vi "STAGE+mono+counter_edit13.vi"() -> ()   [LabVIEW 2017]
panel:
  out "XY Graph 2":cluster{"X":dbl, "Y":dbl}[](graph)
  out "Numeric 2":i32
  out "Numeric":i32
  out "?":cluster{dbl[], dbl[]}(graph)
  out "XY Graph":cluster{dbl[], dbl[]}(graph)
  out "Slide":u8(slide) max=10 step=10 scale=0.0..10.0
  in  "?":enum32{"DELAY", "COUNTER", "MONO", "PLOT"}(tab)
  out "Final time [ps]":dbl
  out "Current time [ps]":dbl
  out "Initial time [ps]":dbl
  in  "Set this as t0":bool
  in  "Axis":i32=1
  in  "Motor ON":bool
  in  "Motor OFF":bool
  out "Current Position [mm]":dbl
  out "Final Position [mm]":dbl
  in  "Data Points":i32=100
  out "Current Point":i32
  in  "Step Size [um]":i32=10
  in  "Target [mm]":dbl format="%.3f"
  in  "Move":bool
  out "Initial position [mm]":dbl
  in  "GPIB address":string="23"
  in  "Count Mode":u16(ring) items=["A,B for Preset T", "A-B for Preset T", "A+B for Preset T", "A for Preset B"]
  in  "Trigger mode":u16(ring) items=["10 MHz"=0, "Input 2"=2, "Input T"=3]
  in  "Channel A Input":u16(ring)=1 items=["10 MHz", "Input 1"]
  in  "Channel B Input":u16(ring)=2 items=["Input 1"=1, "Input 2"=2]
  in  "Number of Measurements\n to take at one point/ Number of Periods":u16=1 min=1 max=2000 step=1
  in  "Time between measurements\n at one point (s)/Dwell Time":dbl=0.002 min=0.002 max=60.0 step=0.001
  in  "gate A mode (CW:0)":i16(slide) scale=0.0..2.0 scale format="%.2f"
  out "Counts":i32
  in  "Integrating time, 10^-7 sec":dbl=10000000.0
  out "Mono port":T1(ring)
  out "Time delay":u32=450000 min=1
  out "Serial":u32=12345
  in  "Step size":dbl=10.0 min=0.0
  in  "Scan to":i32=4000
  in  "Scan from":i32=2600
  out "Current wavelength":dbl
  out "Grt#":u8=1 min=1 max=3 step=1
  in  "?":bool
  out "Groove/mm":u32=1200
  out "Blaze (nm)":u32=300
  in  "Array":dbl[](array[numeric])
  out "Timeout 2":bool
  in  "?":bool
  out "Timeout":bool
  in  "Collect Data!":bool
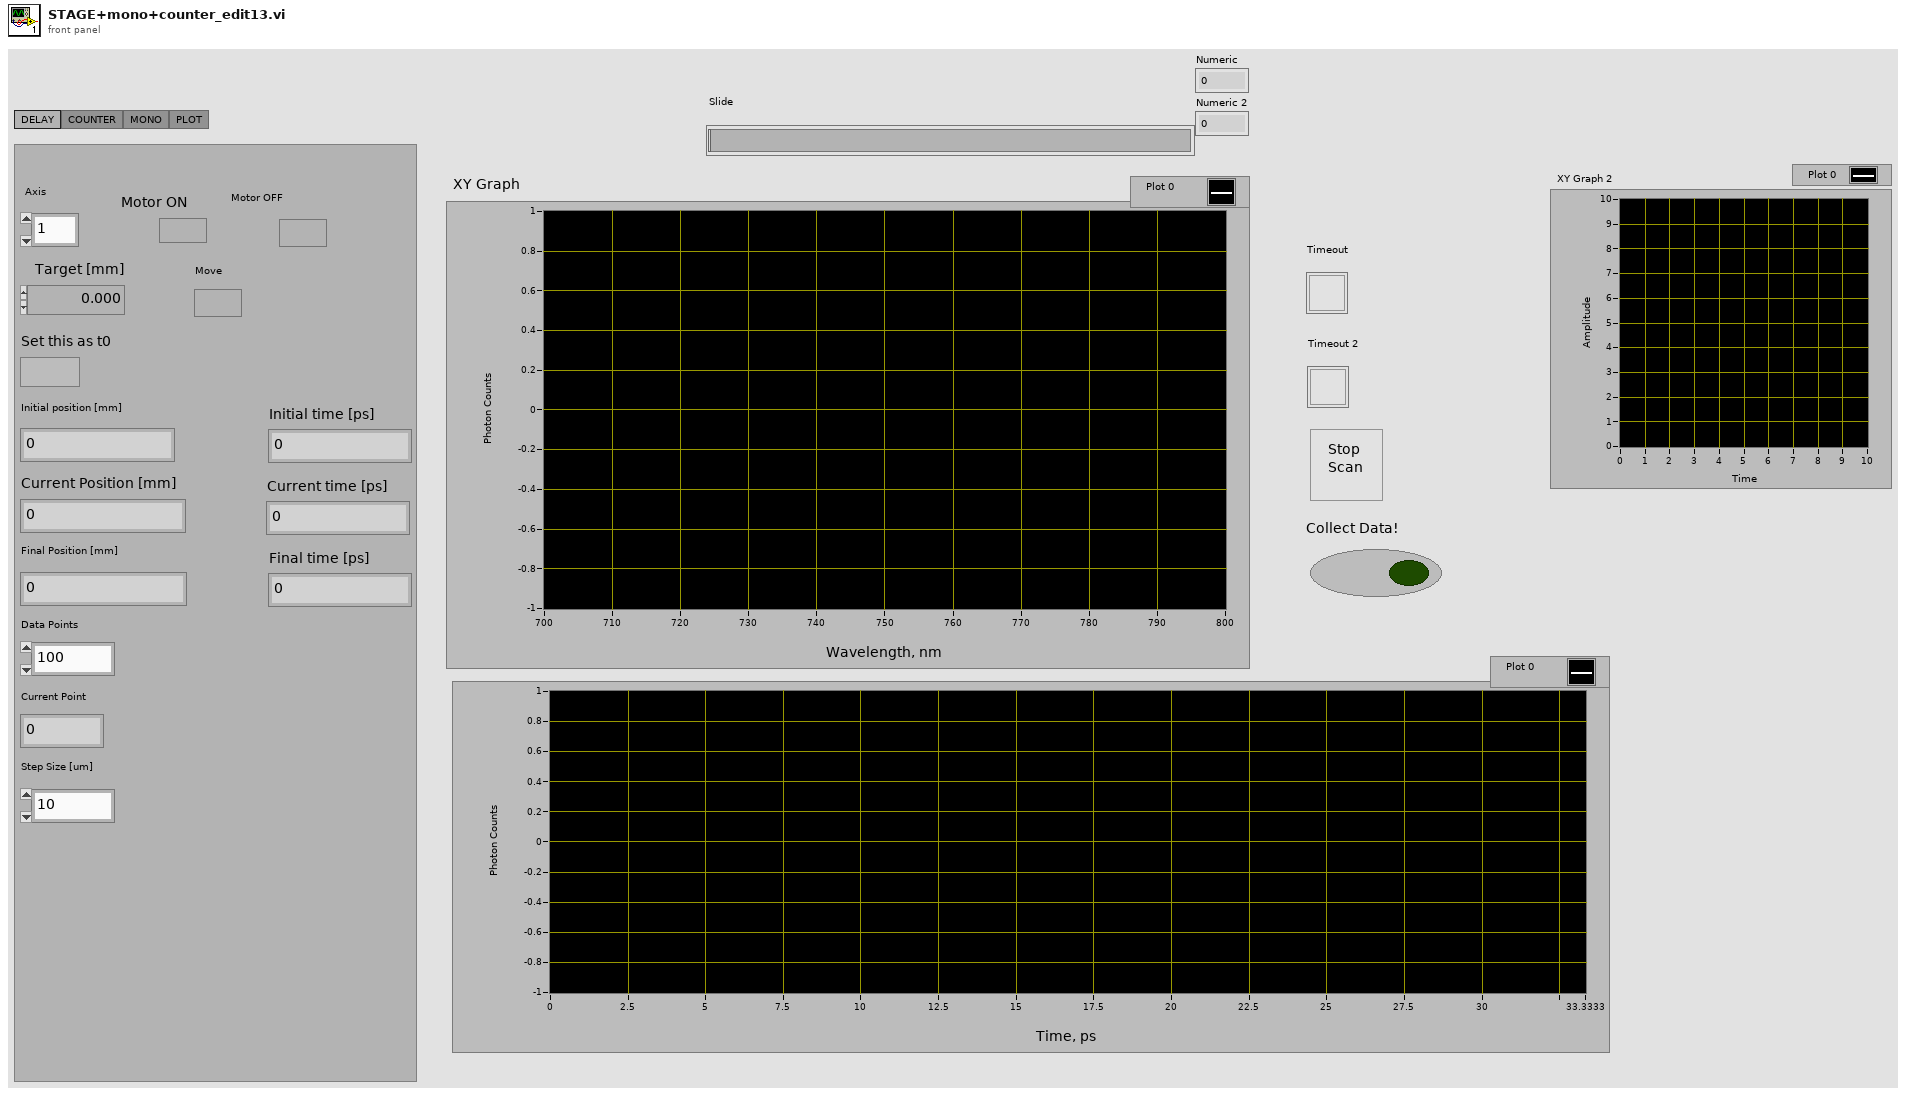
[diagram p1: front panel]
types:
  T1 = enum8{"COM 1", "COM 2", "COM 3", "COM 4", "COM 5", "COM 6", "COM 7", "COM 8", "COM 9"}
  T2 = cluster{"input XON/XOFF":bool, "input HW Handshake":bool, "input alt HW HShk":bool, "output XON/XOFF":bool, "output HW Handshake":bool, "output alt HW HShk":bool, "XOFF byte":u8, "XON byte":u8, "parity error byte":u16}
  T3 = enum16{"no parity", "odd parity", "even parity", "mark parity", "space parity"}
  T4 = cluster{"Y[0]":dbl, "Y[1]":dbl, "Y[2]":dbl, "Y[3]":dbl, "Y[4]":dbl, "Y[5]":dbl, "Y[6]":dbl, "Y[7]":dbl, "Y[8]":dbl}
  T5 = typedef "NI_Matrix.lvlib/RealMatrix.ctl" = dbl[][]
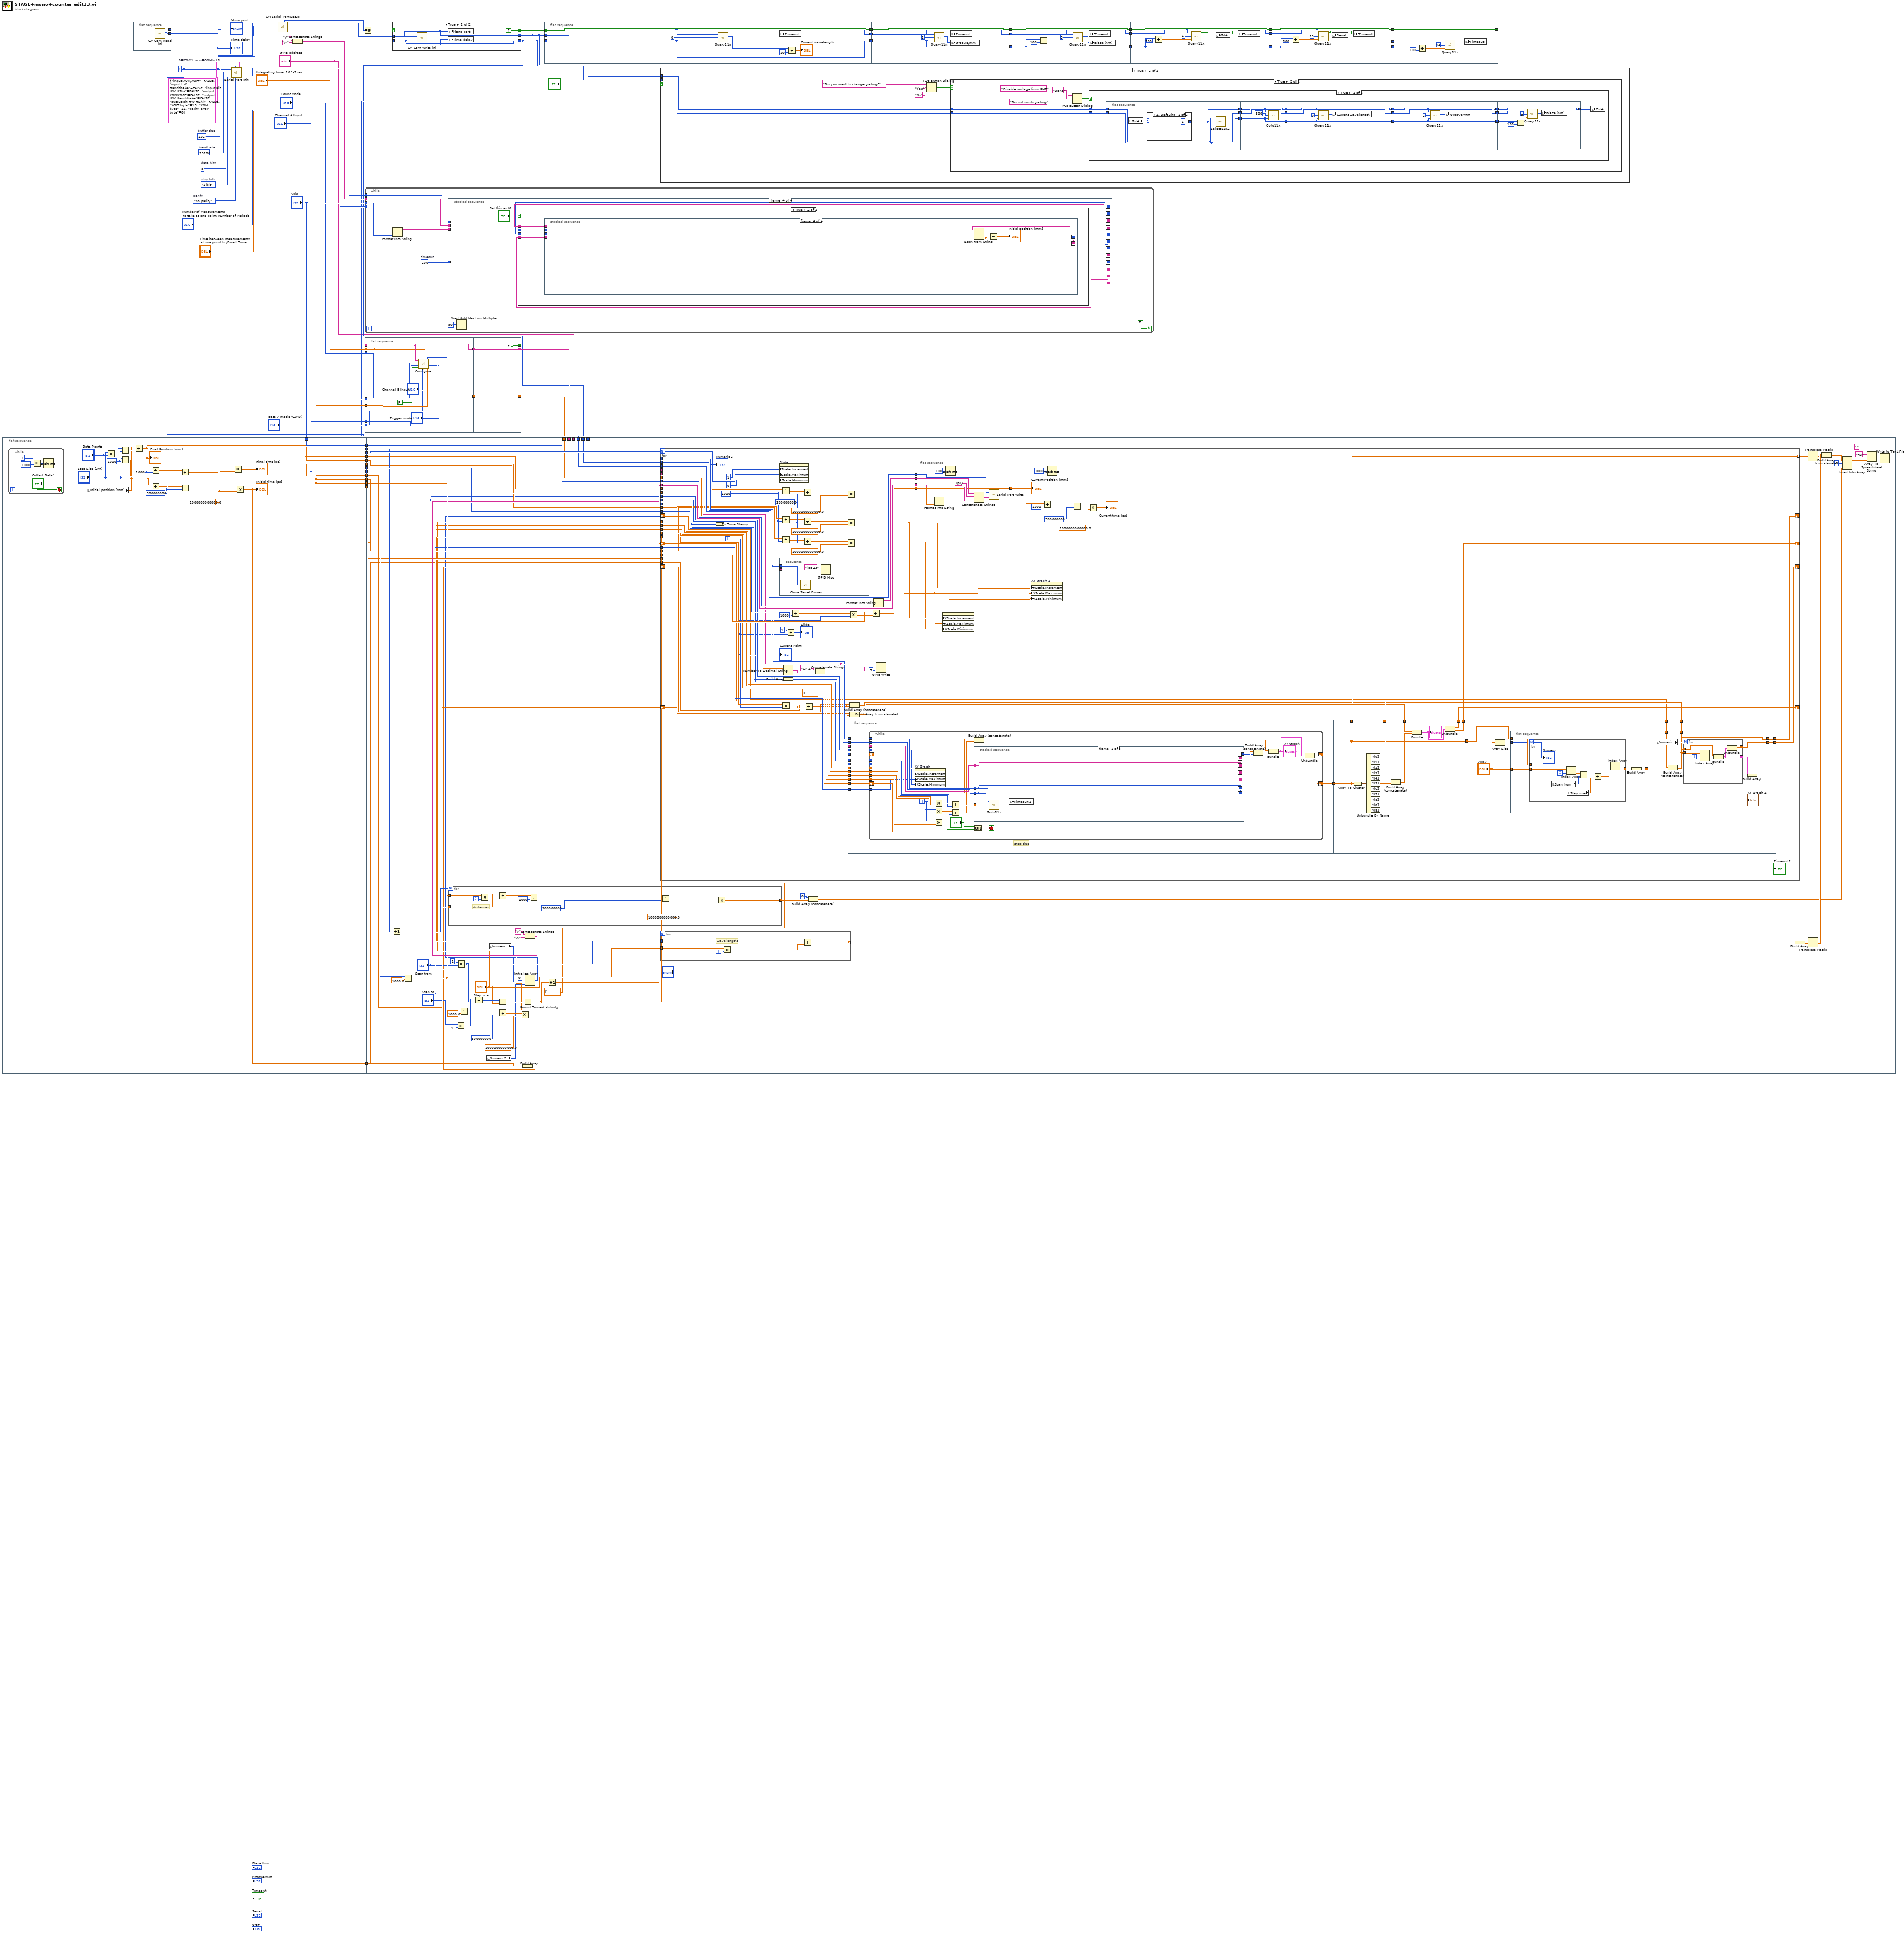
[diagram p0: block diagram]
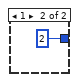
[diagram p5: hidden frame]
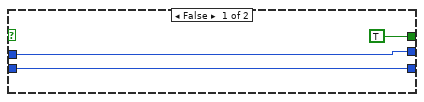
[diagram p6: hidden frame]
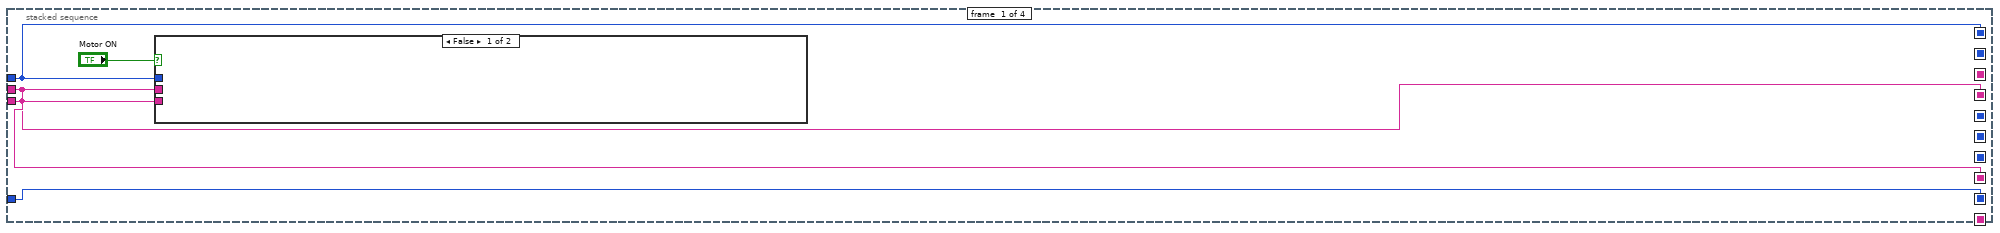
[diagram p7: hidden frame]
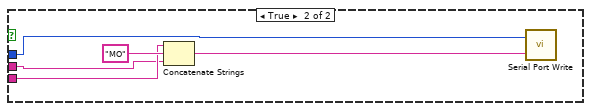
[diagram p8: hidden frame]
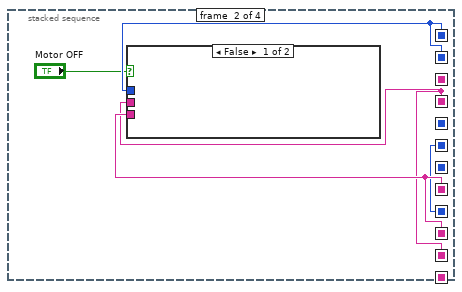
[diagram p9: hidden frame]
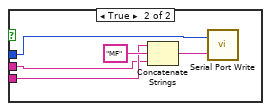
[diagram p10: hidden frame]
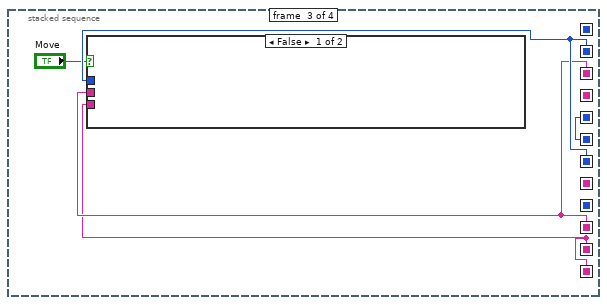
[diagram p11: hidden frame]
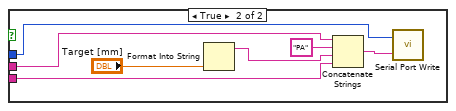
[diagram p12: hidden frame]
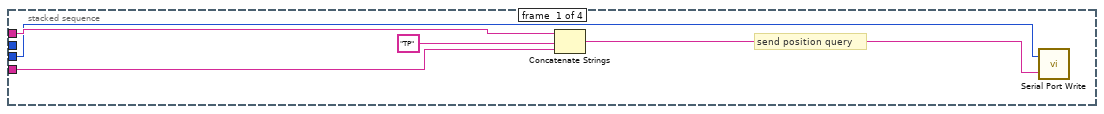
[diagram p14: hidden frame]
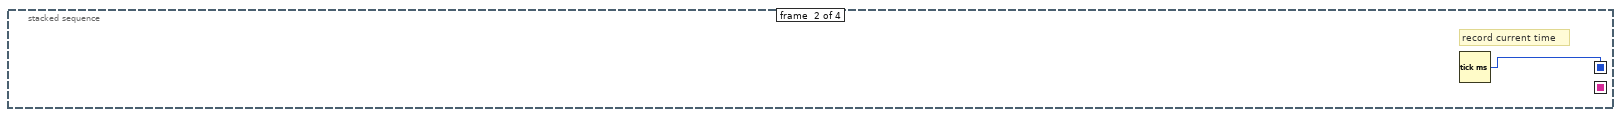
[diagram p15: hidden frame]
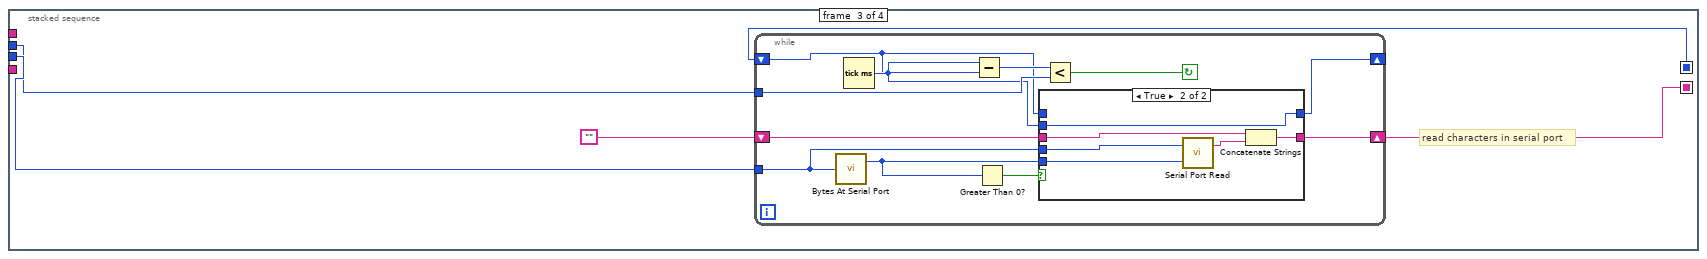
[diagram p16: hidden frame]
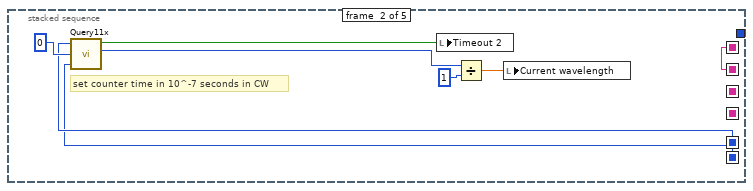
[diagram p18: hidden frame]
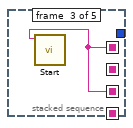
[diagram p19: hidden frame]
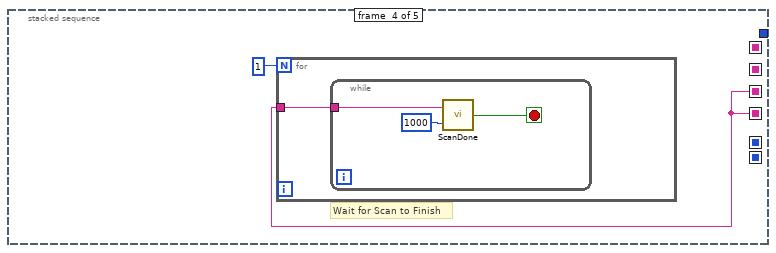
[diagram p20: hidden frame]
diagram:
  w55 = u32 19200  # baud rate
  w54 = u16 8  # data bits
  w53 = enum16{"1 bit", "1.5 bits", "2 bits"}."1 bit"  # stop bits
  w57 = T3."no parity"  # parity
  w52 = 4  # 0=COM1 so n=COM(n+1)
  w56 = u16 1024  # buffer size
  n1 = flat-sequence {
    tunnel: ["Data Points"] -> w61
    tunnel: "Axis" -> [w83]
    tunnel: [w75] -> w60
    tunnel: [w83] -> w59
    tunnel: ["Step Size [um]"] -> w12
    tunnel: [w75] -> w11
    tunnel: ["Step Size [um]"] -> w10
    tunnel: ["Data Points"] -> w9
    tunnel: [w75] -> w8
    tunnel: [w74] -> w7
    tunnel: [w75] -> w4
    tunnel: [w74] -> w3
    tunnel: [w77] -> w2
    tunnel: [w67] -> w1
    tunnel: w61 -> [w145]
    tunnel: w60 -> [w144]
    tunnel: w59 -> [w143]
    tunnel: w52 -> [w139]
    tunnel: w16 -> [w138]
    tunnel: w15 -> [w137]
    tunnel: w14 -> [w136]
    tunnel: "GPIB address" -> [w135]
    tunnel: w12 -> [w122]
    tunnel: w11 -> [w120]
    tunnel: w10 -> [w119]
    tunnel: w9 -> [w117]
    tunnel: w8 -> [w110]
    tunnel: w7 -> [w109]
    tunnel: w6 -> [w108]
    tunnel: w4 -> [w106]
    tunnel: w3 -> [w105]
    tunnel: w2 -> [w104]
    tunnel: w1 -> [w102]
    frame #0 {
      n2 = while {
        stop <- "Collect Data!" stop-if-true
        n3 = Multiply(x=1, y=1000) -> (x*y=w65:i32)
        n4 = Wait (ms)(milliseconds to wait=w65) -> ()  [unwired: 1 out]
      }
    }
    frame #1 {
      w68 = 1000000000000.0
      w73 = 1000
      w76 = 300000000
      w78 = 1000
      n5 = local read "Initial position [mm]"() -> (w75:dbl)
      n6 = Multiply(x="Step Size [um]", y="Data Points") -> (x*y=w82:i32)
      n7 = Divide(x=w82, y=w78) -> (x/y=w81:dbl)
      n8 = Divide(x="Step Size [um]", y=w78) -> (x/y=w77:dbl)
      n9 = Add(x=w75, y=w81) -> (x+y=w74:dbl)
      "Final Position [mm]" <- w74
      n10 = Divide(x=w74, y=w73) -> (x/y=w72:dbl)
      n11 = Divide(x=w75, y=w73) -> (x/y=w71:dbl)
      n12 = Divide(x=w72, y=w76) -> (x/y=w69:dbl)
      n13 = Divide(x=w71, y=w76) -> (x/y=w70:dbl)
      n14 = Multiply(x=w69, y=w68) -> (x*y=→"Final time [ps]":dbl)
      n15 = Multiply(x=w70, y=w68) -> (x*y=w67:dbl)
      "Initial time [ps]" <- w67
    }
    frame #2 {
      n16 = Increment(x=w117) -> (x+1=w118:i32)
      n17 = Divide(x=w122, y=1000.0) -> (x/y=w96:dbl)
      n18 = for {
        N: w118 -> [_]
        tunnel: w96 -> [w156]
        tunnel: w120 -> [w154]
        tunnel: [w147] -> w116 mode=indexing
        i -> [w155]
        # "distances"
        n19 = Multiply(x=w156, y=w155) -> (x*y=w153:dbl)
        n20 = Add(x=w154, y=w153) -> (x+y=w152:dbl)
        n21 = Divide(x=w152, y=1000) -> (x/y=w146:dbl)
        n22 = Divide(x=w146, y=300000000) -> (x/y=w149:dbl)
        n23 = Multiply(x=w149, y=1000000000000.0) -> (x*y=w147:dbl)
      }
      n24 = Multiply(x="Scan to", y=1) -> (x*y=w103:i32)
      n25 = Multiply(x=1, y="Scan from") -> (x*y=w92:i32)
      n26 = Divide(x=w96, y=1000.0) -> (x/y=w97:dbl)
      n27 = Subtract(x=w103, y=w92) -> (x-y=w130:i32)
      n28 = local read "Numeric 2"() -> (w85:i32)
      n29 = local read "Numeric"() -> (w84:i32)
      n30 = Divide(x=w130, y="Step size") -> (x/y=w129:dbl)
      n31 = Divide(x=w97, y=300000000) -> (x/y=w99:dbl)
      n32 = Multiply(x=w99, y=1000000000000.0) -> (x*y=w95:dbl)
      n33 = Build Array(w102) -> (w89:dbl[])
      n34 = Round Toward -Infinity(1:w129) -> (0:w128:dbl)
      n35 = Concatenate Strings("\r", "\n") -> (w140:string)
      n36 = Initialize Array(0, w84, w85) -> (w87:i32[][])
      n37 = Increment(x=w128) -> (x+1=w91:dbl)
      n38 = for {
        N: w145 -> [w204]
        tunnel: w144 -> [w231]
        tunnel: w119 -> [w227]
        tunnel: w143 -> [w224]
        tunnel: w140 -> [w221]
        tunnel: w139 -> [w222]
        tunnel: w138 -> [w220]
        tunnel: w137 -> [w217]
        tunnel: w136 -> [w219]
        tunnel: w135 -> [w218]
        tunnel: [w169] -> w125 mode=indexing
        tunnel: w92 -> [w212]
        tunnel: "Step size" -> [w211]
        tunnel: w128 -> [w210]
        tunnel: w110 -> [_]
        tunnel: w109 -> [_]
        tunnel: w108 -> [w209]
        tunnel: "Scan to" -> [w208]
        tunnel: "Scan from" -> [w207]
        tunnel: "Step size" -> [w178]
        tunnel: w106 -> [w199]
        tunnel: w105 -> [w197]
        tunnel: w104 -> [w200]
        tunnel: w95 -> [w187]
        shift-right: [w171] -> _
        shift-left: w89 -> [w181]
        shift-right: [w170] -> _
        shift-left: dbl[] [] ("Y") -> [w176]
        tunnel: w102 -> [w205]
        tunnel: "Scan from" -> [w179]
        tunnel: "Step size" -> [w180]
        shift-right: [w168] -> _
        shift-left: w89 -> [w174]
        shift-right: [w166] -> _
        shift-left: w87 -> [w165]
        i -> [w186]
        w198 = 1000
        w201 = 300000000
        n39 = To Time Stamp(1:w212) -> ()  [unwired: 1 out]
        n40 = property on="Slide" class="Slide (strict)"("Scale.Increment"=1, "Scale.Maximum"=w204, "Scale.Minimum"=0) -> ()  [unwired: 2 in, 2 out]
        n41 = stacked-sequence {
          tunnel: w217 -> [w345]
          tunnel: w218 -> [_]
          frame #0 {
            n42 = call <vilib>:"Close Serial Driver.vi"("port number"=w345) -> ()  [unwired: 1 out]
            n43 = GPIB Misc(0:"loc 23" ("command string")) -> ()  [unwired: 1 in, 3 out]
          }
        }
        n44 = Divide(x=w197, y=w198) -> (x/y=w194:dbl)
        n45 = Divide(x=w200, y=w198) -> (x/y=w196:dbl)
        n46 = Divide(x=w199, y=w198) -> (x/y=w195:dbl)
        n47 = Multiply(x=w187, y=w186) -> (x*y=w206:dbl)
        n48 = Number To Decimal String(number=w209) -> (decimal integer string=w215:string)  [unwired: 1 in]
        n49 = Build Array(w179) -> (w183:i32[])
        n50 = Add(x=1, y=w186) -> (x+y=→"Slide":i32)
        n51 = Divide(x=w227, y=1000) -> (x/y=w226:dbl)
        n52 = Divide(x=w194, y=w201) -> (x/y=w188:dbl)
        n53 = Divide(x=w196, y=w201) -> (x/y=w190:dbl)
        n54 = Divide(x=w195, y=w201) -> (x/y=w189:dbl)
        n55 = Add(x=w205, y=w206) -> (x+y=w175:dbl)
        n56 = Concatenate Strings("CP 2,", w215) -> (w213:string)
        n57 = Multiply(x=w188, y=1000000000000.0) -> (x*y=w163:dbl)
        n58 = Multiply(x=w190, y=1000000000000.0) -> (x*y=w164:dbl)
        n59 = Multiply(x=w189, y=1000000000000.0) -> (x*y=w162:dbl)
        n60 = flat-sequence {
          tunnel: w220 -> [w245]
          tunnel: w219 -> [w244]
          tunnel: w217 -> [w243]
          tunnel: w212 -> [w242]
          tunnel: w211 -> [w241]
          tunnel: w210 -> [w240]
          tunnel: w208 -> [w239]
          tunnel: w207 -> [w238]
          tunnel: w183 -> [w237]
          tunnel: dbl[] [] ("Y") -> [w236]
          tunnel: w180 -> [w235]
          tunnel: w179 -> [w234]
          tunnel: w178 -> [w233]
          tunnel: [w232] -> w177
          tunnel: w177 -> [w299]
          tunnel: w176 -> [w306]
          tunnel: [w299] -> w173
          tunnel: w172 -> [w303]
          tunnel: [w301] -> w171
          tunnel: [w300] -> w170
          tunnel: [w299] -> w169
          tunnel: w173 -> [w315]
          tunnel: [w308] -> w168
          tunnel: w167 -> [w309]
          tunnel: w165 -> [w312]
          tunnel: [w310] -> w166
          frame #0 {
            # "step size"
            n61 = while {
              tunnel: w243 -> [w271]
              tunnel: w244 -> [w270]
              tunnel: w245 -> [w266]
              tunnel: w242 -> [w264]
              tunnel: w241 -> [w263]
              tunnel: w240 -> [w262]
              tunnel: w239 -> [w246]
              tunnel: w238 -> [w247]
              tunnel: w233 -> [w248]
              tunnel: w235 -> [w260]
              shift-right: [w255] -> w232
              shift-left: w236 -> [w254]
              shift-right: [w249] -> _
              shift-left: w237 -> [w258]
              tunnel: w234 -> [w252]
              i -> [w261]
              stop <- w269 stop-if-true
              n62 = property on="XY Graph" class="XYGraph (strict)"("XScale.Increment"=w248, "XScale.Maximum"=w246, "XScale.Minimum"=w247) -> ()  [unwired: 2 in, 2 out]
              n63 = Multiply(x=w261, y=w263) -> (x*y=w272:dbl)
              n64 = Multiply(x=w261, y=w260) -> (x*y=w259:dbl)
              n65 = Greater Or Equal?(x=w261, y=w262) -> (x >= y?=w267:bool)
              n66 = Add(x=w272, y=w264) -> (x+y=w265:dbl)
              n67 = Add(x=w259, y=w252) -> (x+y=w257:dbl)
              n68 = Or(x="?", y=w267) -> (x .or. y?=w269:bool)
              n69 = Build Array (concatenate)(w258, w257) -> (w256:dbl[])
              n70 = stacked-sequence {
                seq-local: [w276 _ _ _ _] -> [_ w284 _ _ _]
                seq-local: [w275 _ _ _ _] -> [_ w283 _ _ _]
                seq-local: [w273 _ _ _ _] -> [_ w281 _ _ _]
                seq-local: [_ w281 _ _ _] -> [_ _ w286 _ _]
                seq-local: [_ _ w286 _ _] -> [_ _ _ w287 _]
                seq-local: [_ _ _ w287 _] -> [_ _ _ _ w294]
                tunnel: w265 -> [w277 _ _ _ _]
                tunnel: w271 -> [w276 _ _ _ _]
                tunnel: w270 -> [w275 _ _ _ _]
                tunnel: w266 -> [w273 _ _ _ _]
                tunnel: [_ _ _ _ w293] -> w251
                frame #0 {
                  n71 = call "Goto11x.vi"("time delay"=w275, "WAVELENGTH"=w277, "port number"=w276) -> ("timeout"=w274:bool)  [unwired: 2 out]
                  n72 = local write "Timeout 2"(w274) -> ()
                }
                frame #1 {
                  # "set counter time in 10^-7 seconds in CW"
                  n73 = call "Query11x.vi"("port number"=w284, "QUERY"=0, "time delay"=w283) -> ("timeout"=w282:bool, "STATUS MESSAGE"=w280:u16)  [unwired: 2 out]
                  n74 = local write "Timeout 2"(w282) -> ()
                  n75 = Divide(x=w280, y=1) -> (x/y=w279:dbl)
                  n76 = local write "Current wavelength"(w279) -> ()
                }
                frame #2 {
                  n77 = call "Start.vi"("GPIB Address"=w286) -> ()  [unwired: 9 in]
                }
                frame #3 {
                  # "Wait for Scan to Finish"
                  n78 = for {
                    N: 1 -> [_]
                    tunnel: w287 -> [w289]
                    n79 = while {
                      tunnel: w289 -> [w290]
                      stop <- w292 stop-if-true
                      n80 = call "ScanDone.vi"("Wait (ms)"=1000, "GPIB Address"=w290) -> ("Scan Finished?"=w292:bool)
                    }
                  }
                }
                frame #4 {
                  n81 = call "Read Data.vi"("Channel Number"=0, "GPIB Address"=w294, "Number of Datapoints"=1) -> ("Data"=w295:i32[])
                  n82 = Index Array(array=w295, index=0) -> (element=w293:i32)
                  "Counts" <- w293
                }
              }
              n83 = Build Array (concatenate)(w254, w251) -> (w253:dbl[])
              n84 = Bundle(w256, w253) -> (w250:cluster{dbl[], dbl[]})  [unwired: 1 in]
              "XY Graph" <- w250
              n85 = Unbundle(w250) -> (w249:dbl[], w255:dbl[])
            }
          }
          frame #1 {
            n86 = Array To Cluster(array=w299) -> (cluster=w307:T4)
            n87 = Unbundle By Name(w307) -> ("Y[5]"=w305:dbl)  [unwired: 10 out]
            n88 = Build Array (concatenate)(w306, w305) -> (w304:dbl[])
            n89 = Bundle(w303, w304) -> (w302:cluster{dbl[], dbl[]})  [unwired: 1 in]
            "?" <- w302
            n90 = Unbundle(w302) -> (w301:dbl[], w300:dbl[])
          }
          frame #2 {
            n91 = Array Size(array="Array") -> (size(s)=w313:i32)
            n92 = flat-sequence {
              tunnel: w315 -> [w320]
              tunnel: "Array" -> [w319]
              tunnel: w313 -> [w318]
              tunnel: [w316] -> w311
              tunnel: w312 -> [w337]
              tunnel: w311 -> [w336]
              tunnel: [w334] -> w310
              tunnel: w309 -> [w333]
              tunnel: [w332] -> w308
              frame #0 {
                n93 = for {
                  N: w318 -> [w322]
                  tunnel: w319 -> [w330]
                  tunnel: w320 -> [w324]
                  tunnel: [w321] -> w317
                  i -> [w329]
                  n94 = local read "Scan from"() -> (w327:i32)
                  n95 = Index Array(array=w330, index=w329) -> (element=w328:dbl)
                  n96 = local read "Step size"() -> (w325:dbl)
                  n97 = Subtract(x=w328, y=w327) -> (x-y=w326:dbl)
                  n98 = Divide(x=w326, y=w325) -> (x/y=w323:dbl)
                  n99 = Index Array(array=w324, index=w323) -> (element=w321:dbl)
                  "Numeric" <- w322
                }
                n100 = Build Array(w317) -> (w316:dbl[])
              }
              frame #1 {
                n101 = local read "Numeric"() -> (w335:i32)
                n102 = Build Array (concatenate)(w337, w336) -> (w334:dbl[][])
                n103 = for {
                  N: w335 -> [_]
                  tunnel: w334 -> [w343]
                  tunnel: w333 -> [w341]
                  tunnel: [w340] -> w332
                  tunnel: [w338] -> w331 mode=indexing
                  i -> [w342]
                  n104 = Index Array(array=w343, index (row)=w342) -> (element=w339:dbl[])  [unwired: 1 in]
                  n105 = Bundle(w341, w339) -> (w338:cluster{dbl[], dbl[]})  [unwired: 1 in]
                  n106 = Unbundle(w338) -> (w340:dbl[])  [unwired: 1 out]
                }
                n107 = Build Array(w331) -> ()  [unwired: 1 out]
              }
            }
          }
        }
        n108 = Multiply(x=w226, y=w186) -> (x*y=w230:dbl)
        n109 = Build Array (concatenate)(w174, w175) -> (w167:dbl[])
        n110 = Build Array (concatenate)(w181, w175) -> (w172:dbl[])
        n111 = Add(x=w231, y=w230) -> (x+y=w229:dbl)
        n112 = Format Into String(w224) -> (resulting string=w223:string)  [unwired: 3 in, 1 out]
        n113 = GPIB Write(0:w220, 1:w213, 2:i16 5 ("mode (0)")) -> ()  [unwired: 2 in, 2 out]
        n114 = flat-sequence {
          tunnel: w229 -> [w348]
          tunnel: [w348] -> w225
          tunnel: w221 -> [w350]
          tunnel: w223 -> [w349]
          tunnel: w222 -> [w346]
          tunnel: w225 -> [w359]
          frame #0 {
            n115 = Format Into String(w348) -> (resulting string=w347:string)  [unwired: 3 in, 1 out]
            n116 = Wait (ms)(milliseconds to wait=u32 100) -> ()  [unwired: 1 out]
            n117 = Concatenate Strings(w349, "PA" ("Substring"), w347, w350) -> (w352:string)
            n118 = call <vilib>:"Serial Port Write.vi"("string to write"=w352, "port number"=w346) -> ()  [unwired: 1 out]
          }
          frame #1 {
            n119 = Divide(x=w359, y=1000) -> (x/y=w357:dbl)
            n120 = Wait (ms)(milliseconds to wait=u32 1000) -> ()  [unwired: 1 out]
            n121 = Divide(x=w357, y=300000000) -> (x/y=w356:dbl)
            n122 = Multiply(x=w356, y=1000000000000.0) -> (x*y=→"Current time [ps]":dbl)
            "Current Position [mm]" <- w359
          }
        }
        n123 = property class="XYGraph (strict)"("XScale.Increment"=w164, "XScale.Maximum"=w163, "XScale.Minimum"=w162) -> ()  [unwired: 2 in, 2 out]
        n124 = property on="XY Graph 2" class="XYGraph (strict)"("XScale.Increment"=w164, "XScale.Maximum"=w163, "XScale.Minimum"=w162) -> ()  [unwired: 2 in, 2 out]
        "Current Point" <- w186
        "Numeric 2" <- w204
      }
      n125 = for {
        N: w91 -> [_]
        tunnel: "Step size" -> [w161]
        tunnel: w92 -> [w159]
        tunnel: [w157] -> w90 mode=indexing
        i -> [w160]
        # "wavelengths"
        n126 = Multiply(x=w161, y=w160) -> (x*y=w158:dbl)
        n127 = Add(x=w159, y=w158) -> (x+y=w157:dbl)
      }
      n128 = Build Array (concatenate)(0, w116) -> (w113:dbl[])
      n129 = Build Array(w90) -> (w126:dbl[][])
      n130 = Transpose Matrix(1:w125) -> (0:w123:dbl[][])
      n131 = Transpose Matrix(1:w126) -> (0:w124:dbl[][])
      n132 = Build Array (concatenate)(w124, w123) -> (w112:T5)
      n133 = Insert Into Array(array=w112, index (row)=0, new element=w113) -> (w111:T5)  [unwired: 1 in]
      n134 = Array To Spreadsheet String(delimiter (Tab)=",", array=w111, 3:"%f" ("format string")) -> (spreadsheet string=w127:string)
      n135 = Write to Text File(text=w127) -> ()  [unwired: 3 in, 3 out]
    }
  }
  n136 = flat-sequence {
    tunnel: [w363] -> w30
    tunnel: [w362] -> w29
    frame #0 {
      n137 = call "CM Com Read ini.vi"() -> ("Mono port"=w362:T1, "time delay1"=w363:u32)  [unwired: 7 in]
    }
  }
  n138 = call <vilib>:"Serial Port Init.vi"("flow control etc."=T2 {"input XON/XOFF"=FALSE, "input HW Handshake"=FALSE, "input alt HW HShk"=FALSE, "output XON/XOFF"=FALSE, "output HW Handshake"=FALSE, "output alt HW HShk"=FALSE, "XOFF byte"=13, "XON byte"=11, "parity error byte"=0}, "parity"=w57, "buffer size"=w56, "stop bits"=w53, "data bits"=w54, "baud rate"=w55, "port number"=w52) -> ("error code"=w51:i32)
  n139 = call "CM Serial Port Setup.vi"("COM port"=w29, "time delay"=w30) -> ("time delay1"=w25:u32, "DK port Out"=w26:T1, "error code"=w28:i32)  [unwired: 7 in]
  n140 = Concatenate Strings("\r", "\n") -> (w47:string)
  n141 = Equal To 0?(x=w28) -> (x = 0?=w27:bool)
  n142 = while {
    tunnel: w52 -> [w366]
    tunnel: w47 -> [w367]
    tunnel: w51 -> [_]
    tunnel: "Axis" -> [w364]
    stop <- TRUE continue-if-true
    w365 = u32 200  # timeout
    n143 = Format Into String(w364) -> (resulting string=w368:string)  [unwired: 3 in, 1 out]
    n144 = stacked-sequence {
      seq-local: [w373 _ _ _] -> [_ w384 _ _]
      seq-local: [w372 _ _ _] -> [_ w383 _ _]
      seq-local: [w374 _ _ _] -> [_ w385 _ _]
      seq-local: [w371 _ _ _] -> [_ w381 _ _]
      seq-local: [_ w384 _ _] -> [_ _ w394 _]
      seq-local: [_ w383 _ _] -> [_ _ w393 _]
      seq-local: [_ w385 _ _] -> [_ _ w395 _]
      seq-local: [_ w381 _ _] -> [_ _ w391 _]
      seq-local: [_ _ w394 _] -> [_ _ _ w407]
      seq-local: [_ _ w393 _] -> [_ _ _ w404]
      seq-local: [_ _ w395 _] -> [_ _ _ w406]
      seq-local: [_ _ w391 _] -> [_ _ _ w405]
      tunnel: w368 -> [w373 _ _ _]
      tunnel: w367 -> [w372 _ _ _]
      tunnel: w366 -> [w374 _ _ _]
      tunnel: w365 -> [w371 _ _ _]
      frame #0 {
        n145 = case shown="False" "Motor ON" {
          tunnel: w374 -> [_ w380]
          tunnel: w373 -> [_ w377]
          tunnel: w372 -> [_ w376]
          frame False {
          }
          frame True {
            n146 = Concatenate Strings(w377, "MO" ("Substring"), w376) -> (w378:string)
            n147 = call <vilib>:"Serial Port Write.vi"("string to write"=w378, "port number"=w380) -> ()  [unwired: 1 out]
          }
        }
      }
      frame #1 {
        n148 = case shown="False" "Motor OFF" {
          tunnel: w385 -> [_ w390]
          tunnel: w384 -> [_ w387]
          tunnel: w383 -> [_ w386]
          frame False {
          }
          frame True {
            n149 = Concatenate Strings(w387, "MF" ("Substring"), w386) -> (w388:string)
            n150 = call <vilib>:"Serial Port Write.vi"("string to write"=w388, "port number"=w390) -> ()  [unwired: 1 out]
          }
        }
      }
      frame #2 {
        n151 = case shown="False" "Move" {
          tunnel: w395 -> [_ w402]
          tunnel: w394 -> [_ w399]
          tunnel: w393 -> [_ w398]
          frame False {
          }
          frame True {
            n152 = Format Into String("Target [mm]") -> (resulting string=w396:string)  [unwired: 3 in, 1 out]
            n153 = Concatenate Strings(w399, "PA" ("Substring"), w396, w398) -> (w400:string)
            n154 = call <vilib>:"Serial Port Write.vi"("string to write"=w400, "port number"=w402) -> ()  [unwired: 1 out]
          }
        }
      }
      frame #3 {
        n155 = case shown="True" "Set this as t0" {
          tunnel: w407 -> [_ w411]
          tunnel: w406 -> [_ w410]
          tunnel: w405 -> [_ w409]
          tunnel: w404 -> [_ w408]
          frame False {
          }
          frame True {
            n156 = stacked-sequence {
              seq-local: [_ w417 _ _] -> [_ _ w419 _]
              seq-local: [_ _ w418 _] -> [_ _ _ w444]
              tunnel: w411 -> [w414 _ _ _]
              tunnel: w410 -> [w413 _ w422 _]
              tunnel: w409 -> [_ _ w420 _]
              tunnel: w408 -> [w412 _ _ _]
              frame #0 {
                # "send position query"
                n157 = Concatenate Strings(w414, "TP" ("Substring"), w412) -> (w415:string)
                n158 = call <vilib>:"Serial Port Write.vi"("string to write"=w415, "port number"=w413) -> ()  [unwired: 1 out]
              }
              frame #1 {
                # "record current time"
                n159 = Tick Count (ms)() -> (millisecond timer value=w417:u32)
              }
              frame #2 {
                # "read characters in serial port"
                n160 = while {
                  shift-left: w419 -> [w423]
                  shift-right: [w424] -> _
                  tunnel: w420 -> [w427]
                  shift-left: "" -> [w430]
                  shift-right: [w429] -> w418
                  tunnel: w422 -> [w431]
                  stop <- w426 continue-if-true
                  n161 = call <vilib>:"Bytes At Serial Port.vi"("port number"=w431) -> ("byte count"=w432:u32)  [unwired: 1 out]
                  n162 = Tick Count (ms)() -> (millisecond timer value=w425:u32)
                  n163 = Subtract(x=w425, y=w423) -> (x-y=w428:u32)
                  n164 = Greater Than 0?(x=w432) -> (x > 0?=w433:bool)
                  n165 = case shown="True" w433 {
                    tunnel: w432 -> [_ w441]
                    tunnel: w431 -> [_ w440]
                    tunnel: w430 -> [w435 w438]
                    tunnel: [w435 w437] -> w429
                    tunnel: [w434 w436] -> w424
                    tunnel: w425 -> [_ w436]
                    tunnel: w423 -> [w434 _]
                    frame False {
                    }
                    frame True {
                      n166 = call <vilib>:"Serial Port Read.vi"("requested byte count"=w441, "port number"=w440) -> ("string read"=w439:string)  [unwired: 1 out]
                      n167 = Concatenate Strings(w438, w439) -> (w437:string)
                    }
                  }
                  n168 = Less?(x=w428, y=w427) -> (x < y?=w426:bool)
                }
              }
              frame #3 {
                n169 = Scan From String(input string=w444) -> (output 1=w442:dbl)  [unwired: 4 in, 3 out]
                n170 = Subtract(x=w442, y=w442) -> (x-y=→"Initial position [mm]":dbl)
              }
            }
          }
        }
      }
    }
    n171 = Wait Until Next ms Multiple(millisecond multiple=u32 50) -> ()  [unwired: 1 out]
  }
  n172 = flat-sequence {
    tunnel: "GPIB address" -> [w452]
    tunnel: [w452] -> w31
    tunnel: "Count Mode" -> [w453]
    tunnel: "Number of Measurements\n to take at one point/ Number of Periods" -> [w450]
    tunnel: "Time between measurements\n at one point (s)/Dwell Time" -> [w449]
    tunnel: "Channel A Input" -> [w454]
    tunnel: "gate A mode (CW:0)" -> [w446]
    tunnel: "Integrating time, 10^-7 sec" -> [w445]
    tunnel: [w445] -> w5
    tunnel: w31 -> [w456]
    tunnel: [w456] -> w16
    tunnel: [FALSE] -> _
    tunnel: [w455] -> w6
    tunnel: w5 -> [w455]
    frame #0 {
      n173 = call "Configure.vi"("Dwell Time (s)"=w449, "Channel T Input"="Trigger mode", "Channel B Input"="Channel B Input", "Channel A Input"=w454, "Integrating time, 10^-7 sec"=w445, "gate mode (CW:0)"=w446, "Scan End Mode"=FALSE, "Number of Periods"=w450, "Count Mode"=w453, "GPIB Address"=w452) -> ()
    }
    frame #1 {
    }
  }
  n174 = case shown="True" w27 {
    tunnel: w26 -> [w460 w463]
    tunnel: w25 -> [w459 w462]
    tunnel: [w460 w463] -> w15
    tunnel: [w459 w462] -> w14
    tunnel: [TRUE FALSE] -> w24
    frame False {
    }
    frame True {
      n175 = call "CM Com Write ini.vi"("time delay1"=w463, "Mono port"=w462) -> ()  [unwired: 7 in]
      n176 = local write "Mono port"(w463) -> ()
      n177 = local write "Time delay"(w462) -> ()
    }
  }
  n178 = flat-sequence {
    tunnel: w14 -> [w469]
    tunnel: [w469] -> w46
    tunnel: w15 -> [w471]
    tunnel: [w471] -> w45
    tunnel: w24 -> [w467]
    tunnel: [w467] -> w44
    tunnel: w46 -> [w474]
    tunnel: [w474] -> w43
    tunnel: w45 -> [w476]
    tunnel: [w476] -> w42
    tunnel: w44 -> [w472]
    tunnel: [w472] -> w41
    tunnel: w43 -> [w484]
    tunnel: [w484] -> w40
    tunnel: w42 -> [w481]
    tunnel: [w481] -> w39
    tunnel: w41 -> [w478]
    tunnel: [w478] -> w38
    tunnel: w40 -> [w492]
    tunnel: [w492] -> w37
    tunnel: w39 -> [w489]
    tunnel: [w489] -> w36
    tunnel: w38 -> [w486]
    tunnel: [w486] -> w35
    tunnel: w37 -> [w500]
    tunnel: [w500] -> w34
    tunnel: w36 -> [w497]
    tunnel: [w497] -> w33
    tunnel: w35 -> [w494]
    tunnel: [w494] -> w32
    tunnel: w34 -> [w507]
    tunnel: w33 -> [w504]
    tunnel: [w502] -> _
    tunnel: w32 -> [w502]
    frame #0 {
      n179 = call "Query11x.vi"("port number"=w471, "QUERY"=u16 0, "time delay"=w469) -> ("timeout"=w468:bool, "STATUS MESSAGE"=w466:u16)  [unwired: 2 out]
      n180 = local write "Timeout"(w468) -> ()
      n181 = Divide(x=w466, y=10 ("Numeric")) -> (x/y=→"Current wavelength":dbl)
    }
    frame #1 {
      n182 = call "Query11x.vi"("port number"=w476, "QUERY"=u16 2, "time delay"=w474) -> ("timeout"=w473:bool, "STATUS MESSAGE"=w475:u16)  [unwired: 2 out]
      n183 = local write "Timeout"(w473) -> ()
      n184 = local write "Groove/mm"(w475) -> ()
    }
    frame #2 {
      n185 = Divide(x=w484, y=i16 100 ("device (1)")) -> (x/y=w482:dbl)
      n186 = call "Query11x.vi"("port number"=w481, "QUERY"=u16 3, "time delay"=w482) -> ("timeout"=w479:bool, "STATUS MESSAGE"=w480:u16)  [unwired: 2 out]
      n187 = local write "Timeout"(w479) -> ()
      n188 = local write "Blaze (nm)"(w480) -> ()
    }
    frame #3 {
      n189 = Divide(x=w492, y=i16 100 ("device (1)")) -> (x/y=w490:dbl)
      n190 = call "Query11x.vi"("port number"=w489, "QUERY"=u16 4, "time delay"=w490) -> ("timeout"=w487:bool, "STATUS MESSAGE"=w488:u16)  [unwired: 2 out]
      n191 = local write "Grt#"(w488) -> ()
      n192 = local write "Timeout"(w487) -> ()
    }
    frame #4 {
      n193 = Divide(x=w500, y=i16 100 ("device (1)")) -> (x/y=w498:dbl)
      n194 = call "Query11x.vi"("port number"=w497, "QUERY"=u16 19, "time delay"=w498) -> ("timeout"=w495:bool, "STATUS MESSAGE"=w496:u16)  [unwired: 2 out]
      n195 = local write "Serial"(w496) -> ()
      n196 = local write "Timeout"(w495) -> ()
    }
    frame #5 {
      n197 = Divide(x=w507, y=i16 100 ("device (1)")) -> (x/y=w505:dbl)
      n198 = call "Query11x.vi"("port number"=w504, "QUERY"=u16 14, "time delay"=w505) -> ("timeout"=w503:bool)  [unwired: 3 out]
      n199 = local write "Timeout"(w503) -> ()
    }
  }
  n200 = case shown="True" "?" {
    tunnel: w14 -> [_ w510]
    tunnel: w15 -> [_ w509]
    frame False {
    }
    frame True {
      n201 = Two Button Dialog(message="Do you want to change grating?", 1:"No" ("F button name (\"Cancel\")"), 2:"Yes" ("T button name (\"OK\")")) -> (T button?=w511:bool)
      n202 = case shown="True" w511 {
        tunnel: w510 -> [_ w516]
        tunnel: w509 -> [_ w515]
        frame False {
        }
        frame True {
          n203 = Two Button Dialog(message="Disable voltage from PMT", 1:"Do not swich grating" ("F button name (\"Cancel\")"), 2:"Done" ("T button name (\"OK\")")) -> (T button?=w517:bool)
          n204 = case shown="True" w517 {
            tunnel: w516 -> [_ w535]
            tunnel: w515 -> [_ w534]
            frame False {
            }
            frame True {
              n205 = flat-sequence {
                tunnel: w535 -> [w539]
                tunnel: [w539] -> w532
                tunnel: w534 -> [w538]
                tunnel: [w538] -> w531
                tunnel: [w536] -> w530
                tunnel: w532 -> [w543]
                tunnel: [w543] -> w529
                tunnel: w531 -> [w544]
                tunnel: [w544] -> w528
                tunnel: w530 -> [w542]
                tunnel: [w542] -> w527
                tunnel: w529 -> [w550]
                tunnel: [w550] -> w526
                tunnel: w528 -> [w549]
                tunnel: [w549] -> w525
                tunnel: w527 -> [w547]
                tunnel: [w547] -> w524
                tunnel: w526 -> [w553]
                tunnel: [w553] -> w523
                tunnel: w525 -> [w554]
                tunnel: [w554] -> w522
                tunnel: w524 -> [w551]
                tunnel: [w551] -> w521
                tunnel: w523 -> [w558]
                tunnel: w522 -> [w559]
                tunnel: [w556] -> w533
                tunnel: w521 -> [w556]
                frame #0 {
                  n206 = local read "Grt#"() -> (w537:u8)
                  n207 = case shown="2, Default" w537 {
                    tunnel: [1 2] -> w536
                    frame 2, Default {
                    }
                    frame 1 {
                    }
                  }
                  n208 = call "Select11x2.vi"("time delay"=w539, "NEW GRT?"=w536, "port number"=w538) -> ()  [unwired: 3 out]
                }
                frame #1 {
                  n209 = call "Goto11x.vi"("time delay"=w543, "WAVELENGTH"=u16 300, "port number"=w544) -> ()  [unwired: 3 out]
                }
                frame #2 {
                  n210 = call "Query11x.vi"("port number"=w549, "QUERY"=u16 0, "time delay"=w550) -> ("STATUS MESSAGE"=w546:u16)  [unwired: 3 out]
                  n211 = local write "Current wavelength"(w546) -> ()
                }
                frame #3 {
                  n212 = call "Query11x.vi"("port number"=w554, "QUERY"=u16 2, "time delay"=w553) -> ("STATUS MESSAGE"=w552:u16)  [unwired: 3 out]
                  n213 = local write "Groove/mm"(w552) -> ()
                }
                frame #4 {
                  n214 = Divide(x=w558, y=i16 100 ("device (1)")) -> (x/y=w560:dbl)
                  n215 = call "Query11x.vi"("port number"=w559, "QUERY"=u16 3, "time delay"=w560) -> ("STATUS MESSAGE"=w557:u16)  [unwired: 3 out]
                  n216 = local write "Blaze (nm)"(w557) -> ()
                }
              }
              n217 = local write "Grt#"(w533) -> ()
            }
          }
        }
      }
    }
  }
  "Mono port" <- w29
  "Time delay" <- w30
